vi "rotation.vi"() -> ()   [LabVIEW 2017]
uses:
  <vilib>/Analysis/coordinate.llb/3D Cartesian Coordinate Rotation (Euler) (Array).vi
  <vilib>/Analysis/NI_AALPro.lvlib
panel:
  in  "Euler Angles":cluster{"phi":dbl, "theta":dbl, "psi":dbl} {"psi" min=0.0 max=6.28 step=0.01 format="%.2f"; "theta" min=0.0 max=3.14 step=0.01 format="%.2f"; "phi" min=0.0 max=6.28 step=0.001 format="%.2f"}
  in  "Array":dbl[][](array[numeric])
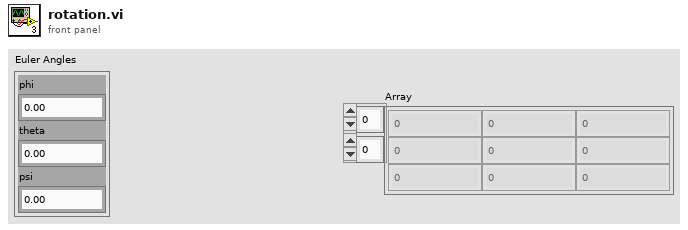
[diagram p1: front panel]
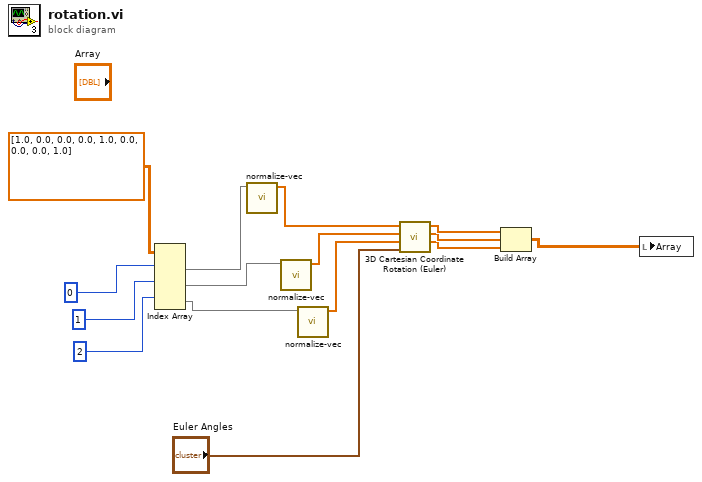
[diagram p0: block diagram]
diagram:
  n1 = Index Array(array=dbl[][] [[1.0, 0.0, 0.0], [0.0, 1.0, 0.0], [0.0, 0.0, 1.0]], index (row) #1=0 ("index (row)"), index (row) #2=1 ("index (row)"), index (row) #3=2 ("index (row)")) -> (element #1=w12:dbl[], element #2=w11:dbl[], element #3=w10:dbl[])  [unwired: 3 in]
  n2 = call "normalize-vec.vi"("Vec Input"=w12) -> ("Array Output"=w9:dbl[])  [unwired: 7 in, 3 out]
  n3 = call "normalize-vec.vi"("Vec Input"=w11) -> ("Array Output"=w8:dbl[])  [unwired: 7 in, 3 out]
  n4 = call "normalize-vec.vi"("Vec Input"=w10) -> ("Array Output"=w7:dbl[])  [unwired: 7 in, 3 out]
  n5 = call-poly <vilib>:"3D Cartesian Coordinate Rotation (Euler).vi"("Euler Angles"="Euler Angles", "Z"=w7, "Y"=w8, "X"=w9) -> ("Z Out"=w3:dbl[], "Y Out"=w4:dbl[], "X Out"=w5:dbl[])  [unwired: 4 in, 1 out]
  n6 = Build Array(w5, w4, w3) -> (w2:dbl[][])
  n7 = local write "Array"(w2) -> ()
